vi "Delete Selected Montage.vi"(8 "error in (no error)":errorcluster, 11 "Data Cluster":T1 {"Settings"."EEG Channels"."16 EEG Channels"."Channel No" step=1}) -> (0 "error out":errorcluster, 3 "Value":i32)   [LabVIEW 2016, in "Settings Editor.lvlib"]
uses:
  Settings Editor.lvlib
  Module Data--cluster.ctl
  Settings--cluster.ctl
  Acquisition/Signal Type--enum.ctl
  Acquisition/Calibration Values--cluster.ctl
  CML Shared/EEG Channel Settings.ctl
  Settings UI Controls.ctl
  Acquisition/Acquisition.lvlib
  CML Shared/CML Shared.lvlib
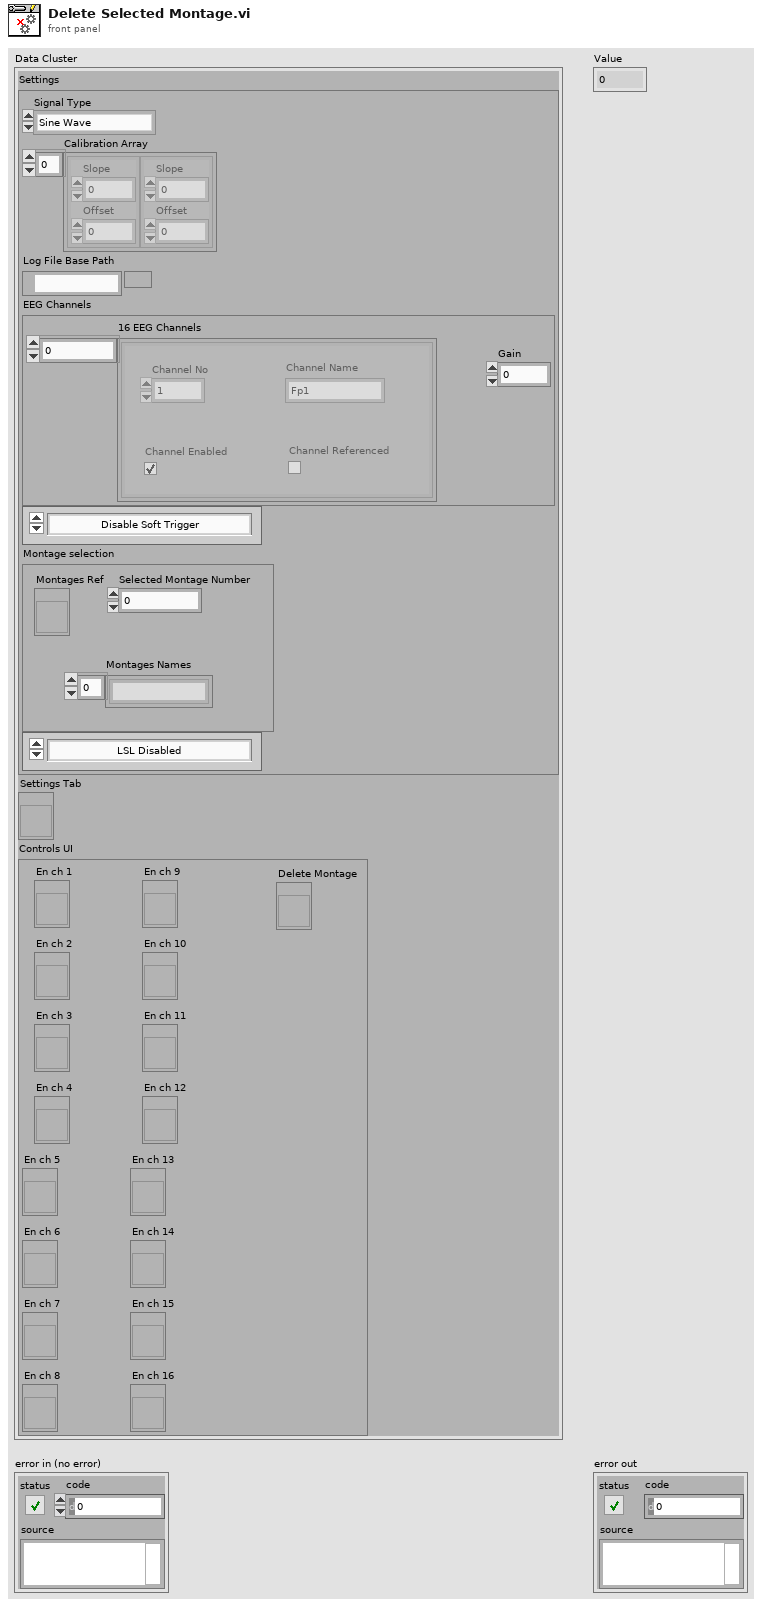
[diagram p1: front panel]
types:
  T1 = typedef "Settings Editor.lvlib/Module Data--cluster.ctl" = cluster{"Settings":T2, "Settings Tab":refnum<vi>, "Controls UI":T6}
  T2 = typedef "Settings Editor.lvlib/Settings--cluster.ctl" = cluster{"Signal Type":T3, "Calibration Array":T4[], "Log File Base Path":path, "EEG Channels":T5, "Soft Trig enum":enum16{"Disable Soft Trigger", "Enable Soft Trigger"}, "Montage selection":cluster{"Montages Ref":refnum<vi>, "Selected Montage Number":u8, "Montages Names":string[]}, "LSL En enum":enum16{"LSL Disabled", "LSL Enabled"}}
  T3 = typedef "Acquisition.lvlib/Signal Type--enum.ctl" = enum16{"Sine Wave", "Square with Noise"}
  T4 = typedef "Acquisition.lvlib/Calibration Values--cluster.ctl" = cluster{"Slope":dbl, "Offset":dbl}
  T5 = typedef "CML Shared.lvlib/EEG Channel Settings.ctl" = cluster{"16 EEG Channels":cluster{"Channel Name":string, "Channel No":u8, "Channel Enabled":bool, "Channel Referenced":bool}[], "Gain":u8}
  T6 = typedef "Settings Editor.lvlib/Settings UI Controls.ctl" = cluster{"En ch 1":refnum<vi>, "En ch 2":refnum<vi>, "En ch 3":refnum<vi>, "En ch 4":refnum<vi>, "En ch 5":refnum<vi>, "En ch 6":refnum<vi>, "En ch 7":refnum<vi>, "En ch 8":refnum<vi>, "En ch 9":refnum<vi>, "En ch 10":refnum<vi>, "En ch 11":refnum<vi>, "En ch 12":refnum<vi>, "En ch 13":refnum<vi>, "En ch 14":refnum<vi>, "En ch 15":refnum<vi>, "En ch 16":refnum<vi>, "Delete Montage":refnum<vi>}
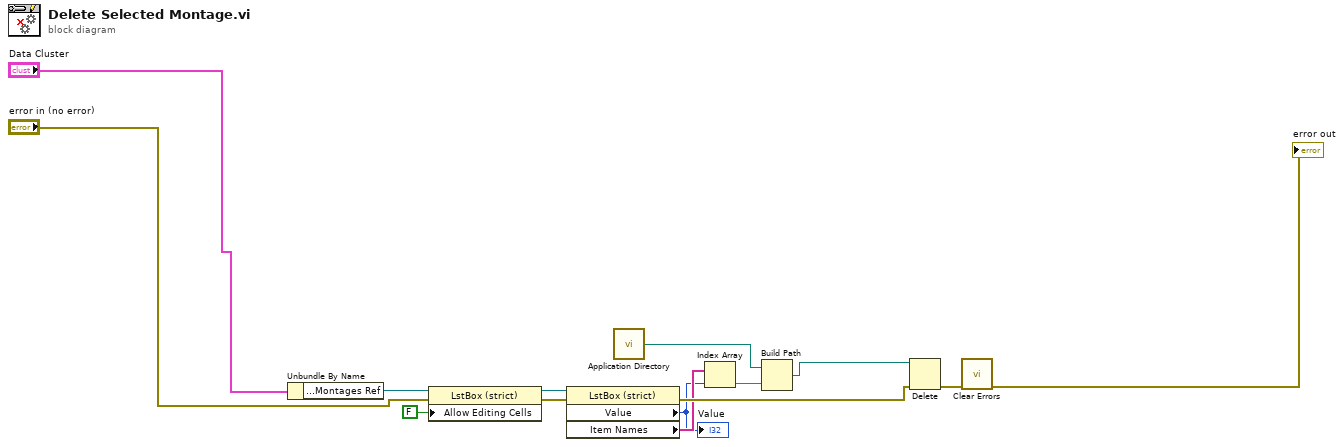
[diagram p0: block diagram]
diagram:
  n1 = Unbundle By Name("Data Cluster") -> ("Settings.Montage selection.Montages Ref"=w6:refnum<vi>)
  n2 = property class="LstBox (strict)"(reference=w6, error in="error in (no error)", "Allow Editing Cells"=FALSE) -> (reference out=w4:refnum<vi>, error out=w11:errorcluster)
  n3 = property class="LstBox (strict)"(reference=w4, error in=w11) -> (error out=w10:errorcluster, "Value"=w2:i32, "Item Names"=w3:string[])  [unwired: 1 out]
  "Value" <- w2
  n4 = call <vilib>:"Application Directory.vi"() -> ("Application Directory"=w1:path)
  n5 = Index Array(array=w3, index=w2) -> (element=w7:string)
  n6 = Build Path(base path=w1, name or relative path=w7) -> (appended path=w9:path)
  n7 = Delete(path (use dialog)=w9, error in=w10) -> (error out=w13:errorcluster)  [unwired: 3 in, 2 out]
  n8 = call <vilib>:"Clear Errors.vi"("error in (no error)"=w13) -> ("error out"=→"error out":errorcluster)  [unwired: 5 in, 1 out]
